vi "质控启动整机或单模块流程对话框.vi"() -> (0 "确定启动":bool, 1 "启动模块":T1, 2 "直接启动":bool, 3 "常规启动":bool)   [LabVIEW 2016, in "质控单元.lvlib"]
uses:
  <vilib>/Utility/miscctls.llb/LVPointTypeDef.ctl
panel:
  in  "整机启动":bool
  in  "取消":bool
  in  "单独启动":bool
  # "请选择启动模式"
  # "单独启动：分参数启动，可先启动某一参数，成功后任意时间\n                  再次进入该界面只能选择其他参数启动 。"
  # "整机启动：整机选参数同时启动，当前测量完成前再次进入该\n                  界面后无法再启动流程。"
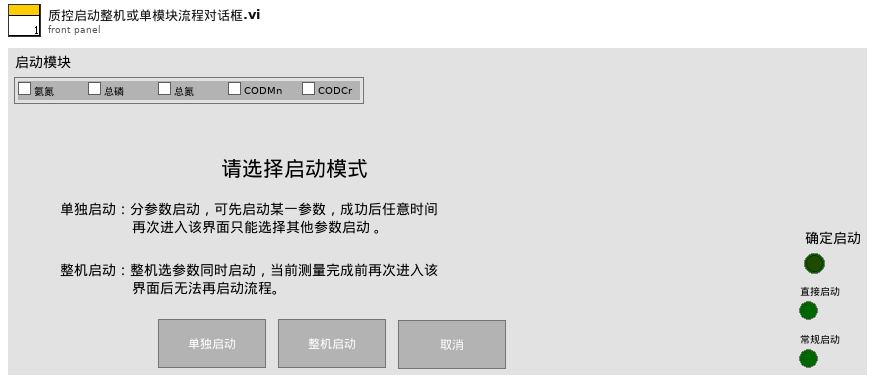
[diagram p1: front panel]
types:
  T1 = cluster{"氨氮":bool, "总磷":bool, "总氮":bool, "CODMn":bool, "CODCr":bool}
  T2 = enum8{"Enabled", "Disabled", "Disabled and Grayed Out"}
  T3 = typedef "LVPointTypeDef.ctl" = cluster{"Horizontal":i16, "Vertical":i16}
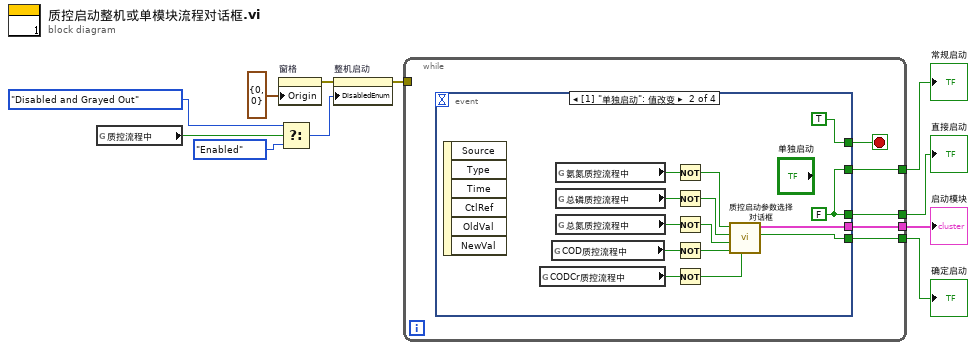
[diagram p0: block diagram]
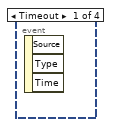
[diagram p2: hidden frame]
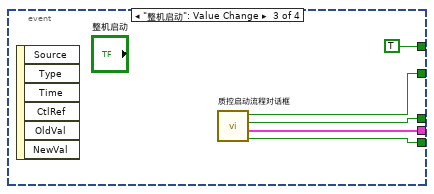
[diagram p3: hidden frame]
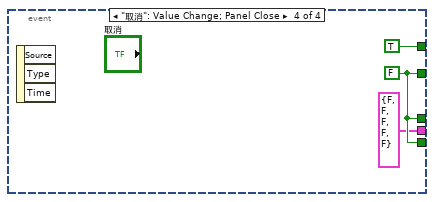
[diagram p4: hidden frame]
diagram:
  n1 = global read "质控测完标志全局 1.vi" "质控流程中"() -> (w3:bool)
  n2 = property on="窗格" class="Pane"("Origin"=T3 {"Horizontal"=0, "Vertical"=0} ("原点")) -> (error out=w1:errorcluster)  [unwired: 2 in, 1 out]
  n3 = Select(t=T2."Disabled and Grayed Out" ("禁用"), s=w3, f=T2."Enabled" ("禁用")) -> (s? t:f=w6:T2)
  n4 = property on="整机启动" class="Bool"(error in=w1, "DisabledEnum"=w6) -> (error out=w2:errorcluster)  [unwired: 1 in, 1 out]
  n5 = while {
    tunnel: [w15] -> w11
    tunnel: [w14] -> w10
    tunnel: [w13] -> w8
    tunnel: [w12] -> w9
    tunnel: w2 -> [_]
    stop <- w16 stop-if-true
    n6 = event shown="[1] \"单独启动\": 值改变" {
      selector: _ -> [_ _ _ _]
      dyn-events: _ -> [_ _ _ _]
      timeout: _ -> [_ _ _ _]
      tunnel: [_ TRUE ("确定") TRUE ("确定") TRUE ("确定")] -> w16
      tunnel: [_ w27 w34 w37] -> w15
      tunnel: [_ w27 w33 w37] -> w14
      tunnel: [_ w29 w32 T1 {"氨氮"=FALSE, "总磷"=FALSE, "总氮"=FALSE, "CODMn"=FALSE, "CODCr"=FALSE} ("启动模块")] -> w13
      tunnel: [_ w28 w31 w37] -> w12
      event Timeout {
        n7 = event-data() -> ()  [unwired: 1 in, 3 out]
      }
      event "单独启动": Value Change {
        w27 = FALSE ("确定")
        n8 = event-data() -> ()  [unwired: 1 in, 6 out]
        n9 = global read "质控测完标志全局 1.vi" "CODCr质控流程中"() -> (w22:bool)
        n10 = global read "质控测完标志全局 1.vi" "COD质控流程中"() -> (w23:bool)
        n11 = global read "质控测完标志全局 1.vi" "氨氮质控流程中"() -> (w26:bool)
        n12 = global read "质控测完标志全局 1.vi" "总磷质控流程中"() -> (w25:bool)
        n13 = global read "质控测完标志全局 1.vi" "总氮质控流程中"() -> (w24:bool)
        n14 = Not(x=w26) -> (.not. x?=w21:bool)
        n15 = Not(x=w25) -> (.not. x?=w20:bool)
        n16 = Not(x=w24) -> (.not. x?=w19:bool)
        n17 = Not(x=w23) -> (.not. x?=w18:bool)
        n18 = Not(x=w22) -> (.not. x?=w17:bool)
        n19 = call "质控启动参数选择对话框.vi"("CODCr"=w17, "CODMn"=w18, "总氮"=w19, "总磷"=w20, "氨氮"=w21) -> ("确定启动"=w28:bool, "启动模块"=w29:T1)  [unwired: 4 in, 1 out]
      }
      event "整机启动": Value Change {
        n20 = event-data() -> ()  [unwired: 1 in, 6 out]
        n21 = call "质控启动流程对话框.vi"() -> ("确定启动"=w31:bool, "启动模块"=w32:T1, "直接启动"=w33:bool, "常规启动"=w34:bool)  [unwired: 8 in]
      }
      event "取消": Value Change; Panel Close {
        w37 = FALSE ("确定")
        n22 = event-data() -> ()  [unwired: 1 in, 3 out]
      }
    }
  }
  "常规启动" <- w11
  "直接启动" <- w10
  "确定启动" <- w9
  "启动模块" <- w8
